vi "Main VERSION 1.1.vi"() -> ()   [LabVIEW 2017]
uses:
  <vilib>/Math Plots/3D Math Plots/3D Surface/3D Surface XCtrl/3D Surface.xctl
  <vilib>/Math Plots/3D Math Plots/3D Surface/3D Surface Datatype/3D Surface Datatype.lvclass
  CSV Reader Inputs.ctl
  Frequency_Type.ctl
  Measurement_Type.ctl
  Digital Channel Selector.ctl
  State.ctl
  Data.ctl
  <vilib>/Platform/TimedLoop/XDataNode/timing_clust.ctl
  <vilib>/Platform/TimedLoop/XDataNode/nitl_modes.ctl
  <vilib>/Platform/TimedLoop/XDataNode/wakeup.ctl
  <vilib>/addons/Control Design/_Model Construction/Data Typedefs.llb/CD DtoC Conversion Method.ctl
  <vilib>/imath/engines/lvmath2/RunTimeEngine/Managers/WorkSpace/UID Generator.vi
  <vilib>/imath/engines/lvmath2/RunTimeEngine/BuiltInFunctions/zpk_to_tf/NIMS_zpk_to_tf.vi
  <vilib>/imath/engines/lvmath2/RunTimeEngine/RunTimeType/NIMS_RunTimeType_From StrictType (excl LVString).vi
  <instcachedir>/0/NIMS_RunTimeType_From StrictType (excl LVString)_DC56D72BB6B948F98D63F1A957D87C42.lvgen/NIMS_RunTimeType_From StrictType (excl LVString)_DC56D72BB6B948F98D63F1A957D87C42_000.vi
  <vilib>/imath/engines/lvmath2/RunTimeEngine/ErrorHandling/NIMS_Error From Error Code.vi
  <vilib>/imath/engines/lvmath2/RunTimeEngine/LocalVariableDefStatement/MC_LocalVariableDefStatement_Display.vi
  <vilib>/imath/engines/lvmath2/RunTimeEngine/Managers/SymbolTable/Clear UID.vi
  <vilib>/imath/engines/lvmath2/RunTimeEngine/NodeEndStatement/NIMS_NodeEndStatement_Output.vi
  <instcachedir>/0/NIMS_NodeEndStatement_Output_53EC0D466D134D7ABD903AC30B43404B.lvgen/NIMS_NodeEndStatement_Output_53EC0D466D134D7ABD903AC30B43404B_005.vi
  <vilib>/imath/engines/lvmath2/RunTimeEngine/ErrorHandling/NIMS_Finalize Error.vi
  <vilib>/addons/Control Design/_Model Construction/Model Creation.llb/Model Creation SubVI/cd_Create Transfer Function Model.vi
  <vilib>/addons/Control Design/_Model Construction/Model Information.llb/Model Information SubVIs/cd_Set Names To TF Model.vi
  <vilib>/addons/Control Design/_Utility/Model Viewer.llb/Model Viewer SubVI/cd_Draw Transfer Function Equation (TF).vi
  <vilib>/addons/Control Design/_Time Response Analysis/Time Response.llb/Time Response subVI/cd_Linear Simulation (Transfer Function).vi
  <vilib>/addons/Control Design/_Dynamic Analysis/Dynamic Analysis.llb/Dynamic Analysis subVI/cd_Damping Ratio and Natural Frequency (Transfer Function).vi
  <vilib>/addons/Wavelet Analysis/application.llb/WA Detrend (Waveform).vi
  Program Files (x86)/National Instruments/LabVIEW 2017/vi.lib/addons/System Identification/Data Preprocess.llb/SI Lowpass Filter (SISO Waveform).vi
  <vilib>/addons/Time Series Analysis/Modeling and Prediction.llb/TSA ARMA Modeling (Waveform).vi
  <vilib>/addons/Control Design/_Model Conversions/Continuous and Discrete.llb/Continuous and Discrete SubVI/cd_Convert Discrete to Continuous (TF).vi
  <vilib>/addons/Control Design/_Model Conversions/Model Type.llb/Model Conversion SubVI/cd_Convert Transfer Function to State-Space Model.vi
  <vilib>/addons/Control Design/_Dynamic Analysis/Dynamic Analysis.llb/Dynamic Analysis subVI/cd_Damping Ratio and Natural Frequency (State-Space).vi
  <vilib>/imath/engines/lvmath2/RunTimeEngine/BuiltInFunctions/sort/NIMS_[2o]_sort(RRowV,I32,Str).vi
  <instcachedir>/0/NIMS_[2o]_sort(RRowV,I32,Str)_E84E23B068DF4763991B1E74560868DE.lvgen/NIMS_[2o]_sort(RRowV,I32,Str)_E84E23B068DF4763991B1E74560868DE_000.vi
  <vilib>/imathl/engines/lvmath/Functions/Error Handling/Create Error.vi
  <vilib>/imath/engines/lvmath2/RunTimeEngine/IndexRead/NIMS V(V).vi
  <instcachedir>/0/NIMS V(V)_298D9CB7BFEB42B8BC8D9C3C28AE8C70.lvgen/NIMS V(V)_298D9CB7BFEB42B8BC8D9C3C28AE8C70_000.vi
  <instcachedir>/0/NIMS V(V)_298D9CB7BFEB42B8BC8D9C3C28AE8C70.lvgen/NIMS V(V)_298D9CB7BFEB42B8BC8D9C3C28AE8C70_001.vi
  <vilib>/imath/engines/lvmath2/RunTimeEngine/BitwiseOperatorToken/NIMS_Bitwise_Operator_And.vi
  <instcachedir>/0/NIMS_Bitwise_Operator_And_BF79565AECDF4B89921EA9614C6BB008.lvgen/NIMS_Bitwise_Operator_And_BF79565AECDF4B89921EA9614C6BB008_001.vi
  <vilib>/imath/engines/lvmath2/RunTimeEngine/BuiltInFunctions/imag/NIMS_imag(Complex).vi
  <instcachedir>/0/NIMS_imag(Complex)_3180D40D00C843A49C2B33397F857BF3.lvgen/NIMS_imag(Complex)_3180D40D00C843A49C2B33397F857BF3_002.vi
  <vilib>/imath/engines/lvmath2/RunTimeEngine/BuiltInFunctions/findnz/NIMS_[1o]_findnz(GRowV).vi
  <instcachedir>/0/NIMS_[1o]_findnz(GRowV)_4566141FE5BA40B7B10E18ED0AB78B2D.lvgen/NIMS_[1o]_findnz(GRowV)_4566141FE5BA40B7B10E18ED0AB78B2D_000.vi
  <vilib>/imath/engines/lvmath2/RunTimeEngine/ErrorHandling/NIMS_Create Error From Enums.vi
  <instcachedir>/0/NIMS_NodeEndStatement_Output_53EC0D466D134D7ABD903AC30B43404B.lvgen/NIMS_NodeEndStatement_Output_53EC0D466D134D7ABD903AC30B43404B_000.vi
  <vilib>/addons/Time Series Analysis/Correlation and Spectral Analysis.llb/TSA ARMA Spectrum (Waveform).vi
  <vilib>/imath/engines/lvmath2/RunTimeEngine/RangeToken/NIMS_Range.vi
  <instcachedir>/0/NIMS_Range_8C005833F4504FD4A29AA23D6150121A.lvgen/NIMS_Range_8C005833F4504FD4A29AA23D6150121A_000.vi
  <vilib>/imath/engines/lvmath2/RunTimeSupport/NIMS_Error if Not Equal.vi
  <instcachedir>/0/NIMS_Error if Not Equal_E5646C1EFB50404BB0542B8CFB81CE27.lvgen/NIMS_Error if Not Equal_E5646C1EFB50404BB0542B8CFB81CE27_001.vi
  <instcachedir>/0/NIMS_Error if Not Equal_E5646C1EFB50404BB0542B8CFB81CE27.lvgen/NIMS_Error if Not Equal_E5646C1EFB50404BB0542B8CFB81CE27_000.vi
  <vilib>/imath/engines/lvmath2/RunTimeEngine/IndexRead/NIMS V($).vi
  <instcachedir>/0/NIMS V($)_C593F32C7F6B43C7B1793952E292524F.lvgen/NIMS V($)_C593F32C7F6B43C7B1793952E292524F_001.vi
  <vilib>/imath/engines/lvmath2/RunTimeEngine/IndexReplace/NIMS M(S,$)=V.vi
  <instcachedir>/0/NIMS M(S,$)=V_552265ADF67C4F4FB07E91CD22492551.lvgen/NIMS M(S,$)=V_552265ADF67C4F4FB07E91CD22492551_000.vi
  <vilib>/imath/engines/lvmath2/RunTimeEngine/IndexReplace/NIMS V(S)=S.vi
  <instcachedir>/0/NIMS V(S)=S_EDDEB2B900FD4B108B325BCE58B17C3D.lvgen/NIMS V(S)=S_EDDEB2B900FD4B108B325BCE58B17C3D_000.vi
  <vilib>/imath/engines/lvmath2/RunTimeEngine/IndexReplace/NIMS V(V)=V.vi
  <instcachedir>/0/NIMS V(V)=V_ACB9F458E2974419B362D656D10048D7.lvgen/NIMS V(V)=V_ACB9F458E2974419B362D656D10048D7_000.vi
  <vilib>/imath/engines/lvmath2/RunTimeEngine/IndexRead/NIMS M(V,$).vi
  <instcachedir>/0/NIMS M(V,$)_21A5155762F74C04AE4EA67BEE0D3EF5.lvgen/NIMS M(V,$)_21A5155762F74C04AE4EA67BEE0D3EF5_004.vi
  <instcachedir>/0/NIMS_NodeEndStatement_Output_53EC0D466D134D7ABD903AC30B43404B.lvgen/NIMS_NodeEndStatement_Output_53EC0D466D134D7ABD903AC30B43404B_009.vi
  <instcachedir>/0/NIMS_NodeEndStatement_Output_53EC0D466D134D7ABD903AC30B43404B.lvgen/NIMS_NodeEndStatement_Output_53EC0D466D134D7ABD903AC30B43404B_002.vi
  <instcachedir>/0/NIMS_NodeEndStatement_Output_53EC0D466D134D7ABD903AC30B43404B.lvgen/NIMS_NodeEndStatement_Output_53EC0D466D134D7ABD903AC30B43404B_001.vi
  <vilib>/Math Plots/3D Math Plots/3D Surface/3D Surface Datatype/Public/Plot Helper (Vector).vi
  <vilib>/platform/TimedLoop/XDataNode/XDataNode.xnode
  Program Files (x86)/National Instruments/LabVIEW 2017/vi.lib/addons/System Identification/NI_SysID.lvlib
  <vilib>/addons/_Advanced Signal Processing/NI_AdvSigProcWA.lvlib
  <vilib>/addons/_Advanced Signal Processing/NI_AdvSigProcTSA.lvlib
  <vilib>/addons/Control Design/_Model Construction/NI_LinSys_Model Creation.lvlib
  <vilib>/addons/Control Design/_Model Conversions/NI_CD_Continuous and Discrete.lvlib
  <vilib>/addons/Control Design/_Model Construction/NI_LinSys_Data Typedefs.lvlib
  <vilib>/Analysis/NI_AALBase.lvlib
  <vilib>/addons/Control Design/_Dynamic Analysis/NI_CD_Dynamic Analysis.lvlib
  <vilib>/Platform/TimedLoop/XDataNode/XDNodeRunTimeDep.lvlib
  <vilib>/addons/Control Design/_Model Conversions/NI_CD_Model Type.lvlib
  <vilib>/Analysis/NI_AALPro.lvlib
  <vilib>/addons/Control Design/_Time Response Analysis/NI_CD_Time Response.lvlib
  <vilib>/imath/engines/lvmath2/RunTimeEngine/Managers/SymbolTable/NIMS_WorkSpace.lvlib
  <vilib>/addons/Control Design/_Model Construction/NI_LinSys_Model Information.lvlib
  <vilib>/addons/Control Design/_Utility/NI_CD_Model Viewer.lvlib
  <vilib>/S3DK/PMU Recorder Light/PMU Recorder Light.lvlib
panel:
  in  "Tab Control 3":enum32{"Test", "Simulation"}(tab)
  in  "Terminal ID 2 (Phase Comparison)":dbl
  in  "Test Method":enum16{"Use PRL Data", "Read from CSV File"}(ring)
  in  "CSV Reader Inputs":T1={"Frequency Type"=enum."Frequency", "Measurement Type"=enum."Power", "Digital Channel Selector"=enum."2", "OGE Type"=enum."OGnE", "CSV File Input"=path ""}
  in  "Terminal ID":dbl
  in  "Input Poles":cdb[](array[numeric])
  in  "Input Zeros":cdb[](array[numeric])
  out "Input Transfer Function":picture
  in  "Input Frequency (Hz)":dbl
  in  "Input Damping Ratio (%)":dbl
  in  "Simulation Method":T5(ring)
  out "Poles":cdb[](array[numeric]) format="%.2f"
  out "Damping Ratios (%)":dbl[](array[numeric]) format="%.2f"
  out "Natural Frequencies":dbl[](array[numeric]) format="%.2f"
  in  "Tab Control":enum32{"Data", "Preprocessed Data"}(tab)
  out "Real-time data":waveform(dbl)(graph)={"t0"=timestamp(3467964116.0127993 s since 1904-01-01), "dt"=0.02, "Y"=array[30000 elements]}
  out "Preprocessed data":waveform(dbl)(graph)={"t0"=timestamp(3467964116.0127993 s since 1904-01-01), "dt"=0.2, "Y"=array[3000 elements]}
  in  "Tab Control 2":T6(tab)=enum."Options"
  out "Critical Damping [%]":dbl
  out "Critical Frequency [Hz]":dbl
  out "Estimated Complex Plane":cluster{dbl[], dbl[]}(graph)
  out "Damping ratio evolution":dbl[][](graph)
  in  "Number of critical modes":i32=1
  in  "Length of Spectra [s]":dbl=12.0
  out "Spectrogram":refnum<class "3D Plot Datatype.lvclass">[](xcontrol)
  in  "dB Scale":bool=TRUE
  out "Spectrum":cluster{"f0":dbl, "df":dbl, "S(f)":dbl[]}(graph)={"f0"=0.0, "df"=0.0048828125, "S(f)"=[]}
  out "ARMA Transfer Function":picture
  out "Picture 9":picture
  out "Picture 8":picture
  out "Picture 7":picture
  out "Picture 6":picture
  out "Picture 5":picture
  out "Picture 4":picture
  out "Picture 3":picture
  out "Picture 2":picture
  out "Picture 1":picture
  out "Std of Damping":dbl[](array[numeric])=[3.167813045881809]
  out "Mean Damping [%]":dbl[](array[numeric])=[5.49924934647624]
  out "Frequency[Hz]":dbl[](array[numeric])=[1.626086044993813, 0.5198061588603065, 1.9739015777045272] format="%.4f"
  out "Damping Ratio [%]":dbl[](array[numeric])=[11.530156484123282, 15.381771713903165, 15.639879258359347] format="%.4f"
  out "Complex Poles":cdb[](array[numeric])=[-1.1780360817698377+10.148858009104277i, -0.5023745738423925+3.227170083530164i, -1.9397187258807729+12.249765461704891i] format="%.4f"
  in  "Upper Damping [%]":dbl=20.0
  in  "Lower Damping [%]":dbl
  in  "Upper Frequency [Hz]":dbl=2.0
  in  "Lower Frequency [Hz]":dbl=0.08
  in  "Signal Selection":T7(radio)=enum."Analog"
  in  "Downsampling Ratio":dbl=1.0
  in  "LPF Cut-off Frequency [Hz]":dbl=2.5
  in  "Low-Pass Filter Order":i32=5
  in  "Detrend Cut-off Frequency (Hz)":dbl=0.05
  in  "MA Order":i32=10
  in  "Sampling Frequency (Hz)":dbl=50.0
  in  "AR Order":i32=25
  in  "Parcel Length (Simulation)":i32=30000
  in  "Refresh Rate [s]":i32=10
  in  "Std Threshold":dbl=1.35
  out "Parcel Length (SDK or Simulation)":i32=30000
  in  "Simulate Data?":bool
  out "Simulation":bool
  in  "stop":bool
  # "Simulated Expected Values"
  # "**Must enter CSV file before running"
  # "***Has the ability to shows more than 1 graph based on parameters\n\n- Each row of data (numerical results) equates to 1 mode"
  # "MA\n_______\n\n   AR"
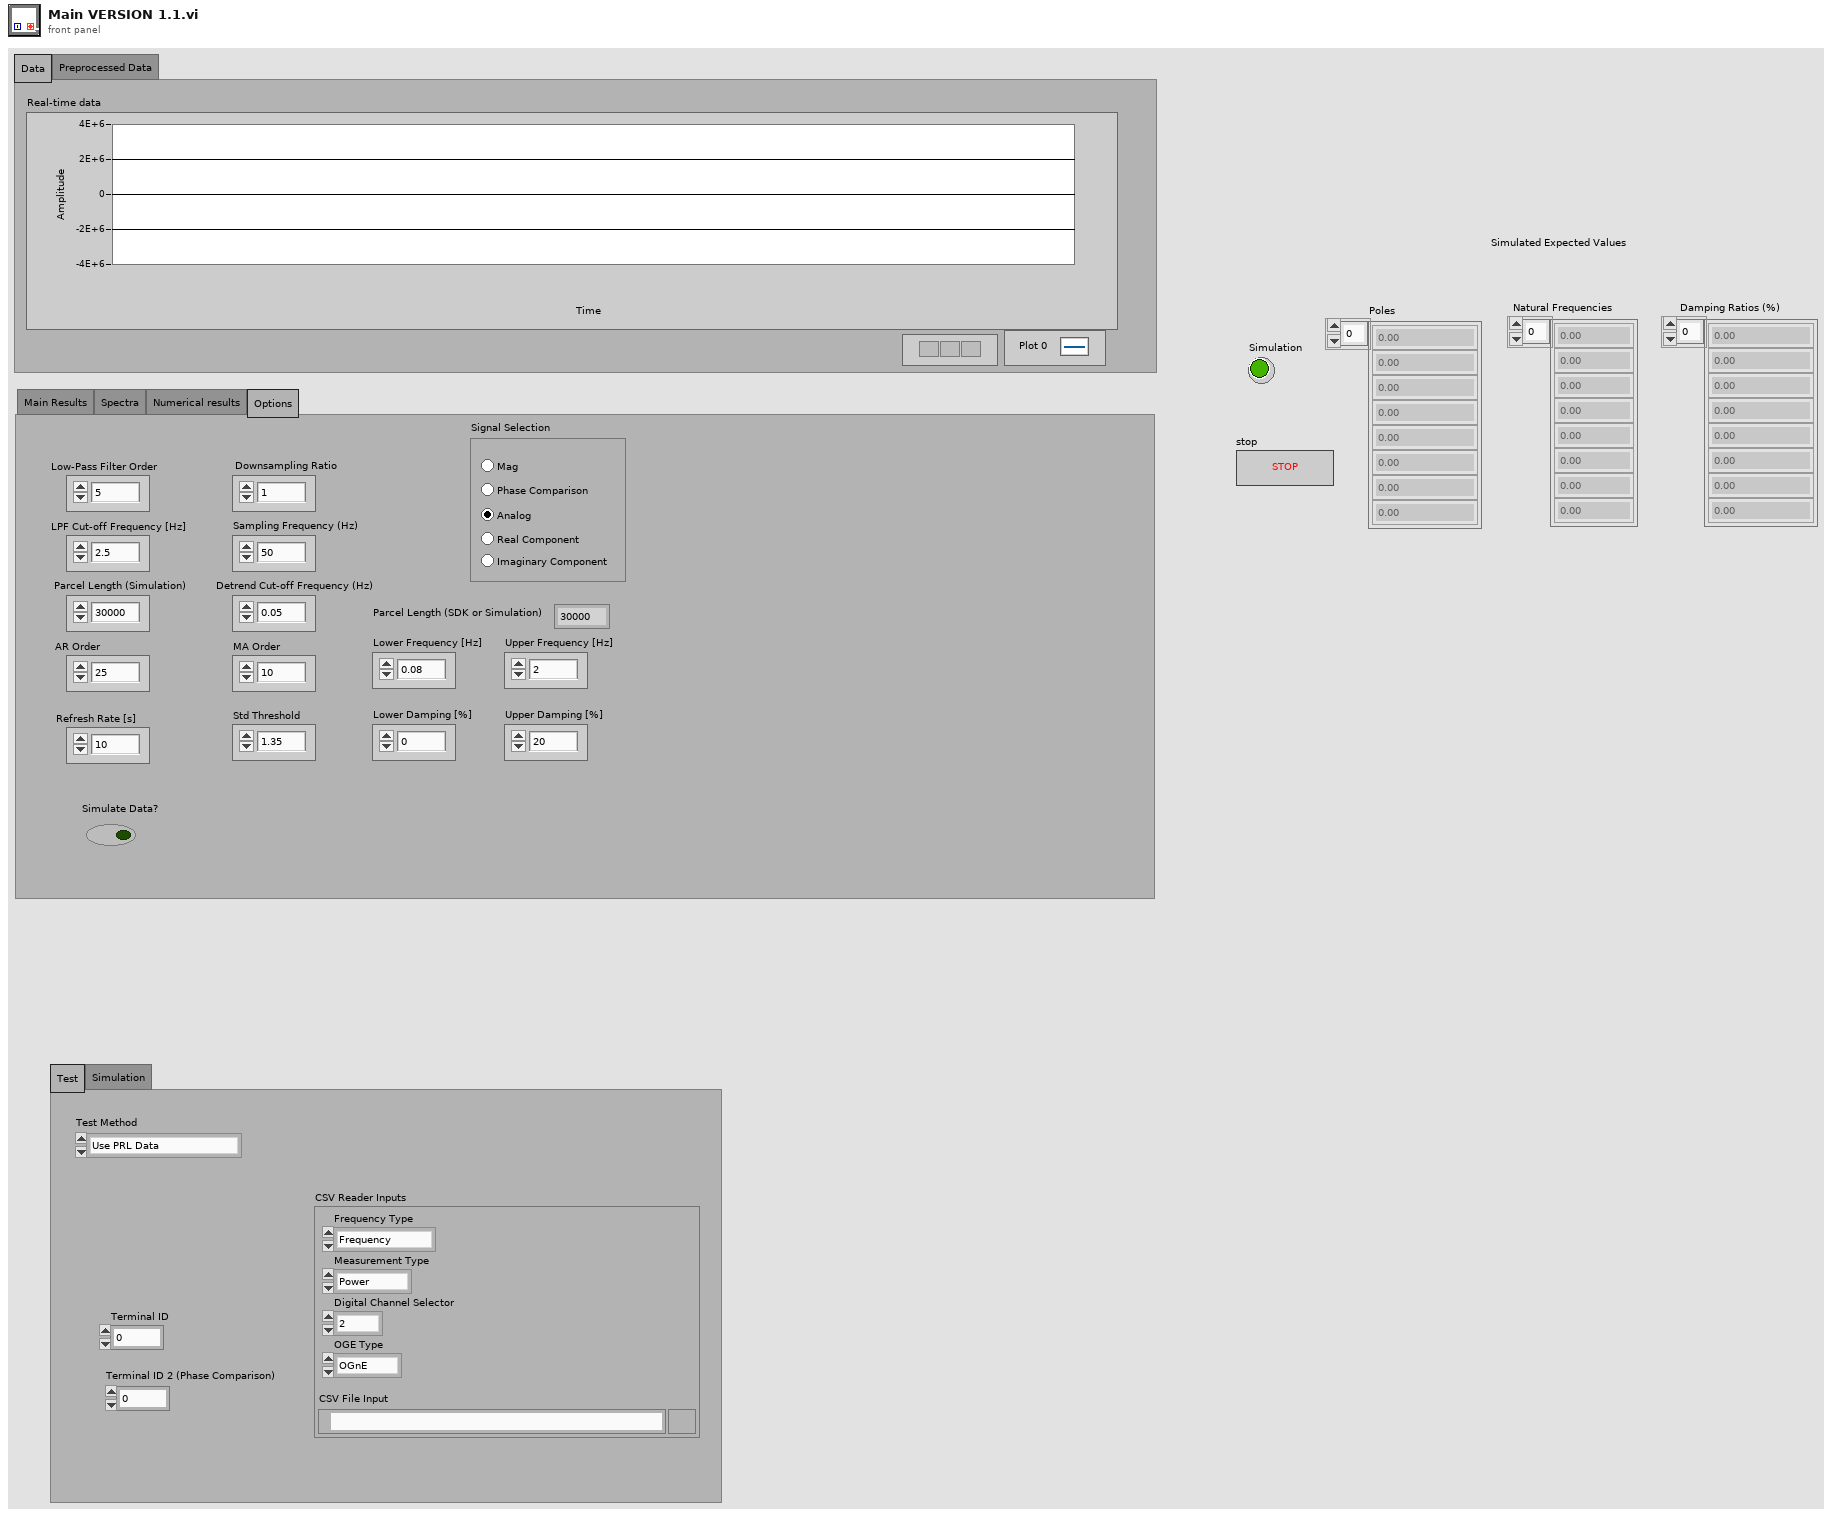
[diagram p1: front panel]
types:
  T1 = typedef "CSV Reader Inputs.ctl" = cluster{"Frequency Type":T2, "Measurement Type":T3, "Digital Channel Selector":T4, "OGE Type":enum16{"WAN OGE", "OGnE"}, "CSV File Input":path}
  T2 = typedef "Frequency_Type.ctl" = enum16{"Frequency", "df/dt"}
  T3 = typedef "Measurement_Type.ctl" = enum16{"Voltage", "Current", "Power"}
  T4 = typedef "Digital Channel Selector.ctl" = enum16{"1", "2", "3"}
  T5 = enum16{"Use Input Frequency/D.R.", "Use Input Poles/Zeroes"}
  T6 = enum32{"Main Results", "Spectra", "Numerical results", "Options"}
  T7 = enum32{"Mag", "Phase", "Analog", "Real Component", "Imaginary Component"}
  T8 = enum8{"Enabled", "Disabled", "Disabled and Grayed Out"}
  T9 = typedef "data.ctl" = cluster{"Waveform":waveform(dbl), "Parcel Length":i32, "AR Order":i32, "Sampling Frequency":dbl, "MA Order ":i32}
  T10 = typedef "State.ctl" = enum16{"Initialize", "Read Real Data", "Read Simulated Data", "Preprocessing", "Compute AR/MA Coeffs", "Get Spectrum"}
  T11 = typedef "XDNodeRunTimeDep.lvlib/timing_clust.ctl" = cluster{"Expected End [f-1]":u64, "Actual End [f-1]":u64, "Finished Late? [f-1]":bool, "Expected End [i-1]":u64, "Actual End [i-1]":u64, "Finished Late? [i-1]":bool, "Expected Start [i]":u64, "Actual Start [i]":u64, "Expected Start [f]":u64, "Actual Start [f]":u64, "Source Name":string, "Structure Name":string, "Period":i64, "Deadline":i64, "Offset":i64, "Start":i64, "Priority":i32, "Timeout":i32, "Mode":T12, "Wakeup Reason":T13, "Error":errorcluster, "Source Type":string, "Secondary Source Type":string, "Global End Time":u64, "Global Start Time":u64, "Frame Duration":u64, "Iteration Duration":u64, "Assigned CPU":i32, "I/O Scan Engine Mode":u32}
  T12 = typedef "XDNodeRunTimeDep.lvlib/nitl_modes.ctl" = enum32{"No Change", "Process missed periods, maintain original phase", "Discard missed periods, maintain original phase", "Process missed periods, ignore original phase", "Discard missed periods, ignore original phase"}
  T13 = typedef "XDNodeRunTimeDep.lvlib/wakeup.ctl" = enum32{"Normal", "Aborted", "Asynchronous wakeup", "Timing source error", "Timed loop error", "Timeout"}
  T14 = typedef "Terminal Data.ctl" = cluster{"Terminal Name":string, "Terminal ID":dbl, "Timestamps":timestamp[], "Phasor Data":cdb[], "Analog Data":dbl[], "Status":dbl[], "Digital Data":dbl[]}
  T15 = typedef "NI_LinSys_Model Typedefs.lvlib/CD Transfer Function Model (MIMO).ctl" = cluster{"properties":T16, "transfer function(s)":T17[][]}
  T16 = typedef "NI_LinSys_Model Typedefs.lvlib/CD General Elements.ctl" = cluster{"Model name":string, "Input names":string[], "Output names":string[], "Input Delays":dbl[], "Output Delays":dbl[], "Sampling Time":dbl, "Notes":string}
  T17 = typedef "NI_LinSys_Model Typedefs.lvlib/CD Transfer Function Model (SISO).ctl" = cluster{"Numerator":dbl[], "Denominator":dbl[], "delay":dbl}
  T18 = typedef "NI_LinSys_Data Typedefs.lvlib/CD MIMO Time Response Data.ctl" = cluster{"Time":dbl[], "Outputs Data":dbl[][][], "States Data":dbl[][][], "plot type":T19}
  T19 = typedef "NI_LinSys_Data Typedefs.lvlib/CD Plot Types Enum.ctl" = enum16{"bode-magnitude", "bode-phase", "nichols", "nyquist", "singular values", "step", "impulse", "initial", "simulation", "nyquist with separation"}
  T20 = typedef "NI_LinSys_Data Typedefs.lvlib/CD DtoC Conversion Method.ctl" = u16
  T21 = typedef "NI_LinSys_Model Typedefs.lvlib/CD State Space Model (MIMO).ctl" = cluster{"properties":T16, "A":dbl[][], "B":dbl[][], "C":dbl[][], "D":dbl[][], "StateNames":string[], "Transport Delay":dbl[][]}
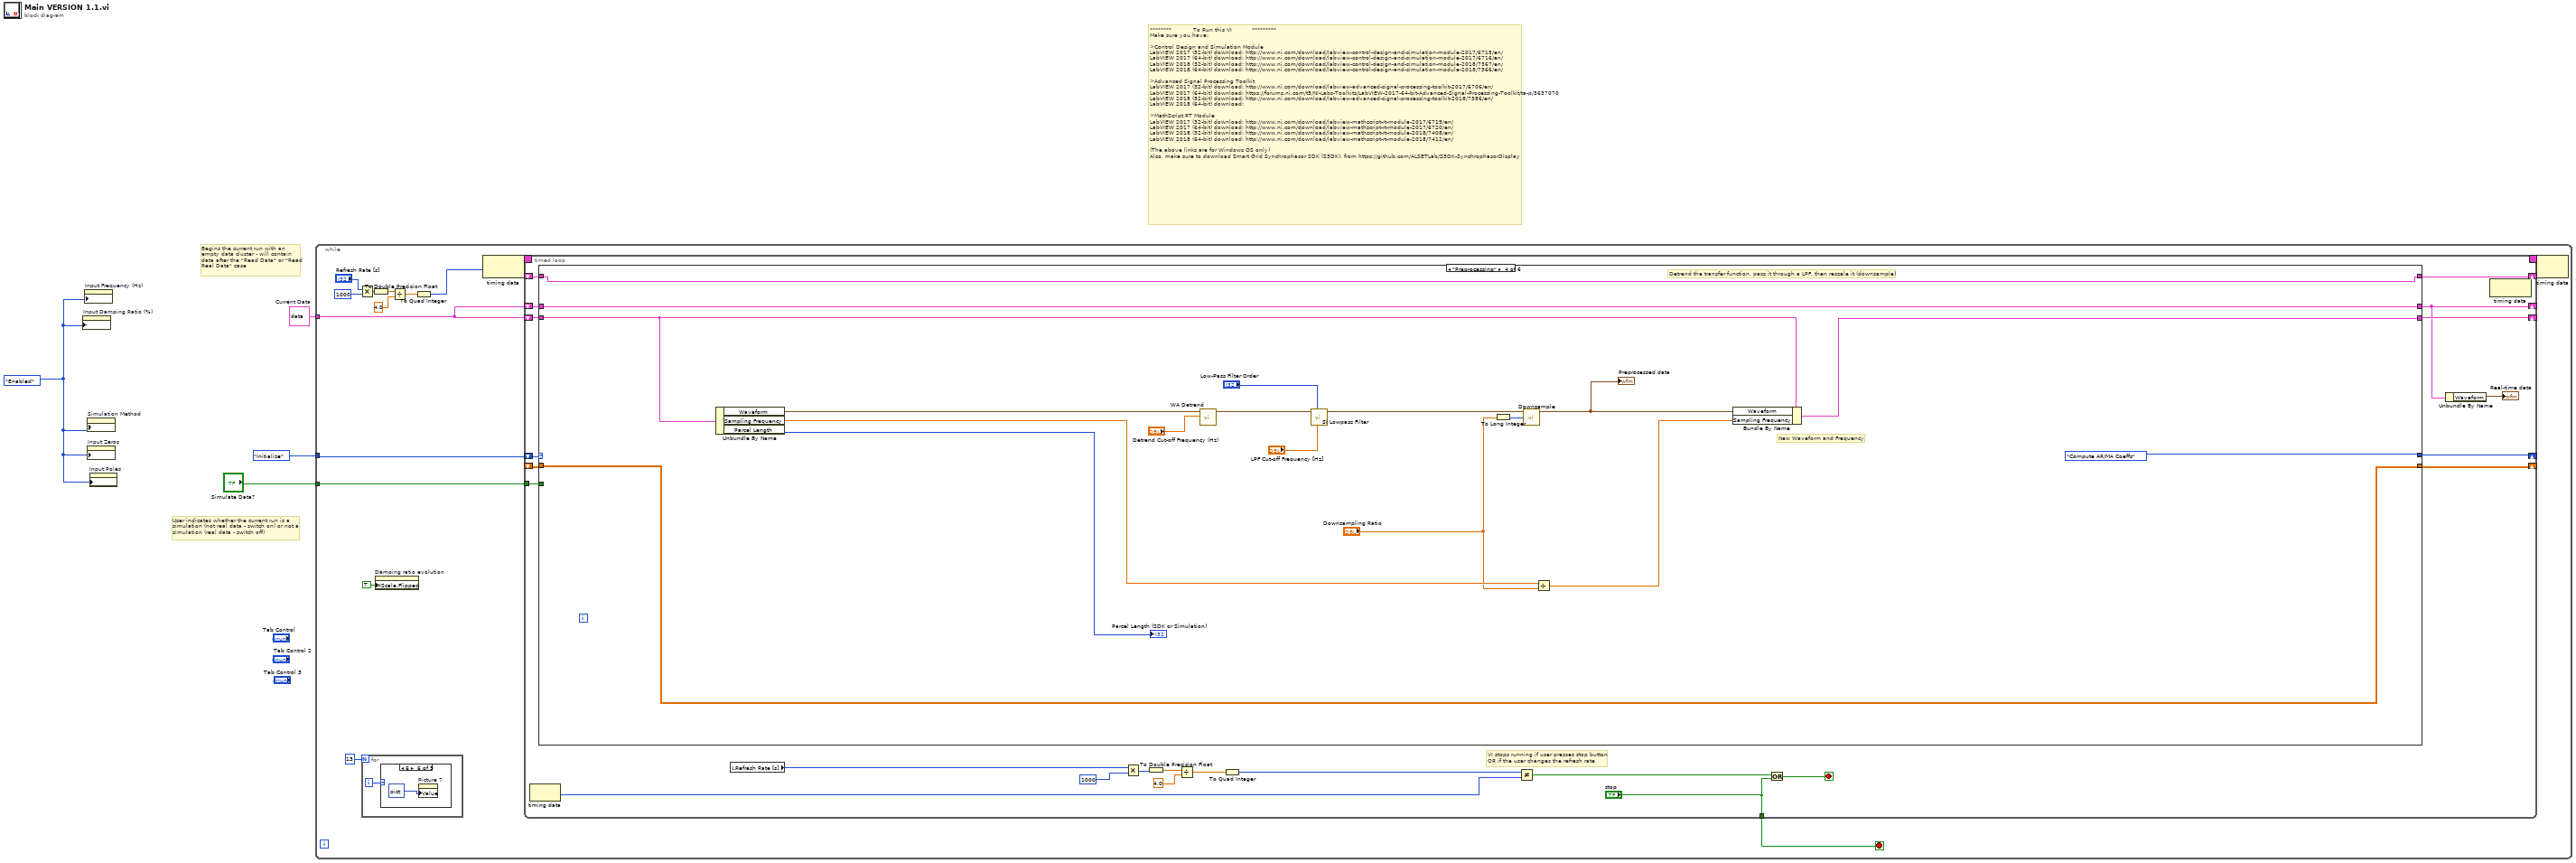
[diagram p0: block diagram]
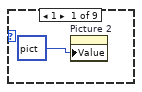
[diagram p2: hidden frame]
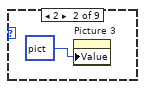
[diagram p3: hidden frame]
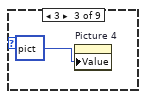
[diagram p4: hidden frame]
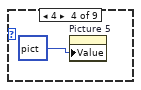
[diagram p5: hidden frame]
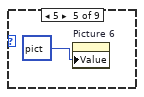
[diagram p6: hidden frame]
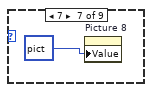
[diagram p7: hidden frame]
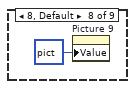
[diagram p8: hidden frame]
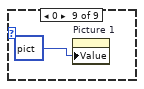
[diagram p9: hidden frame]
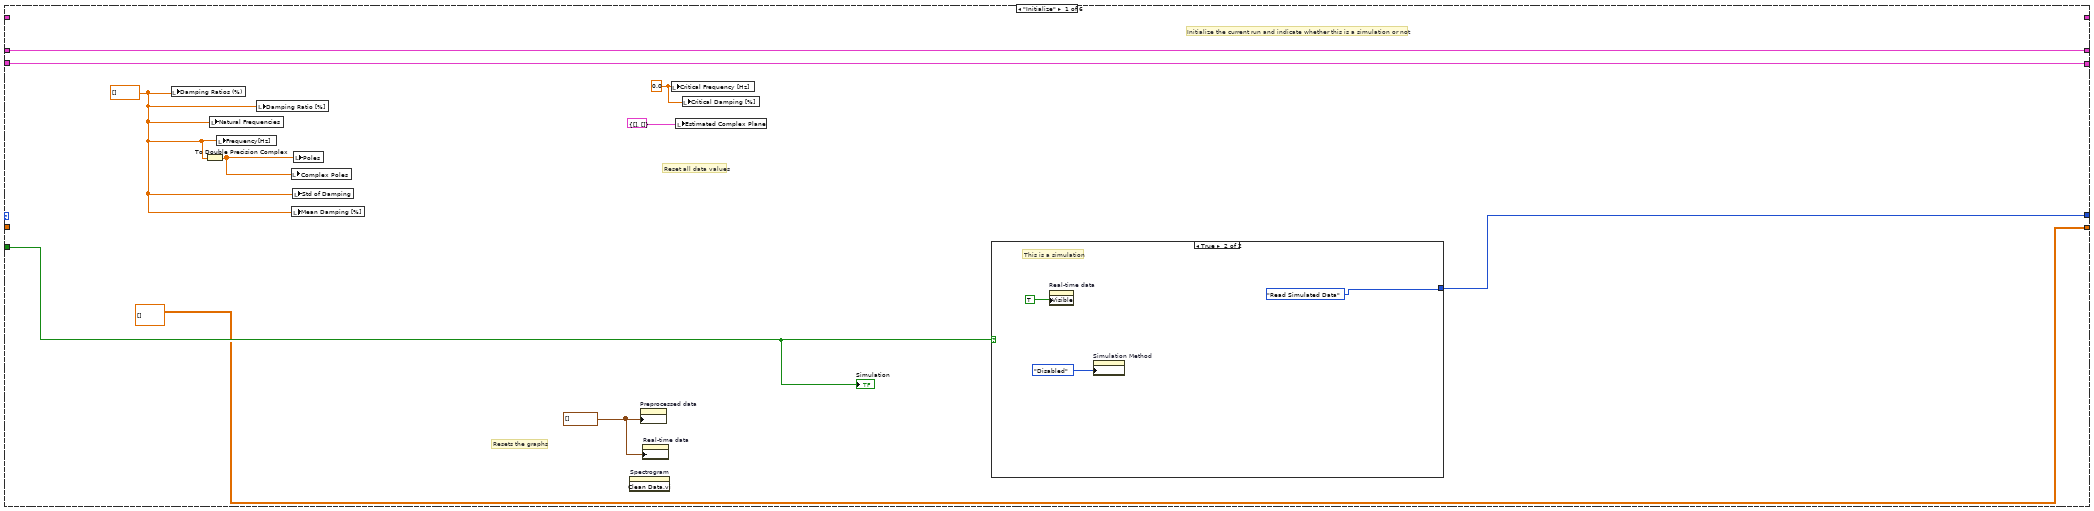
[diagram p10: hidden frame]
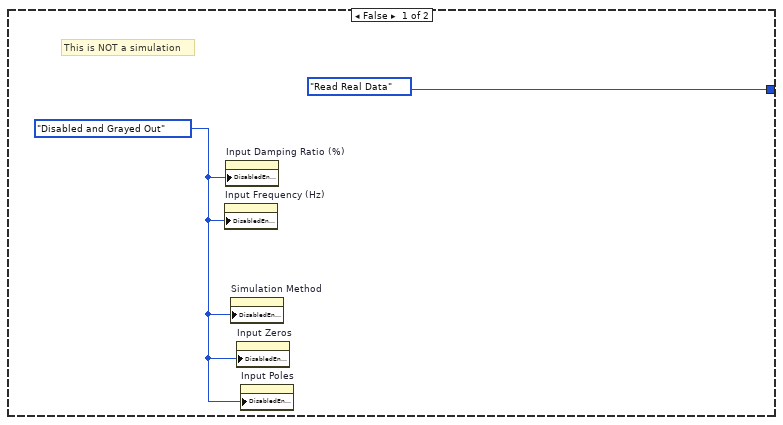
[diagram p11: hidden frame]
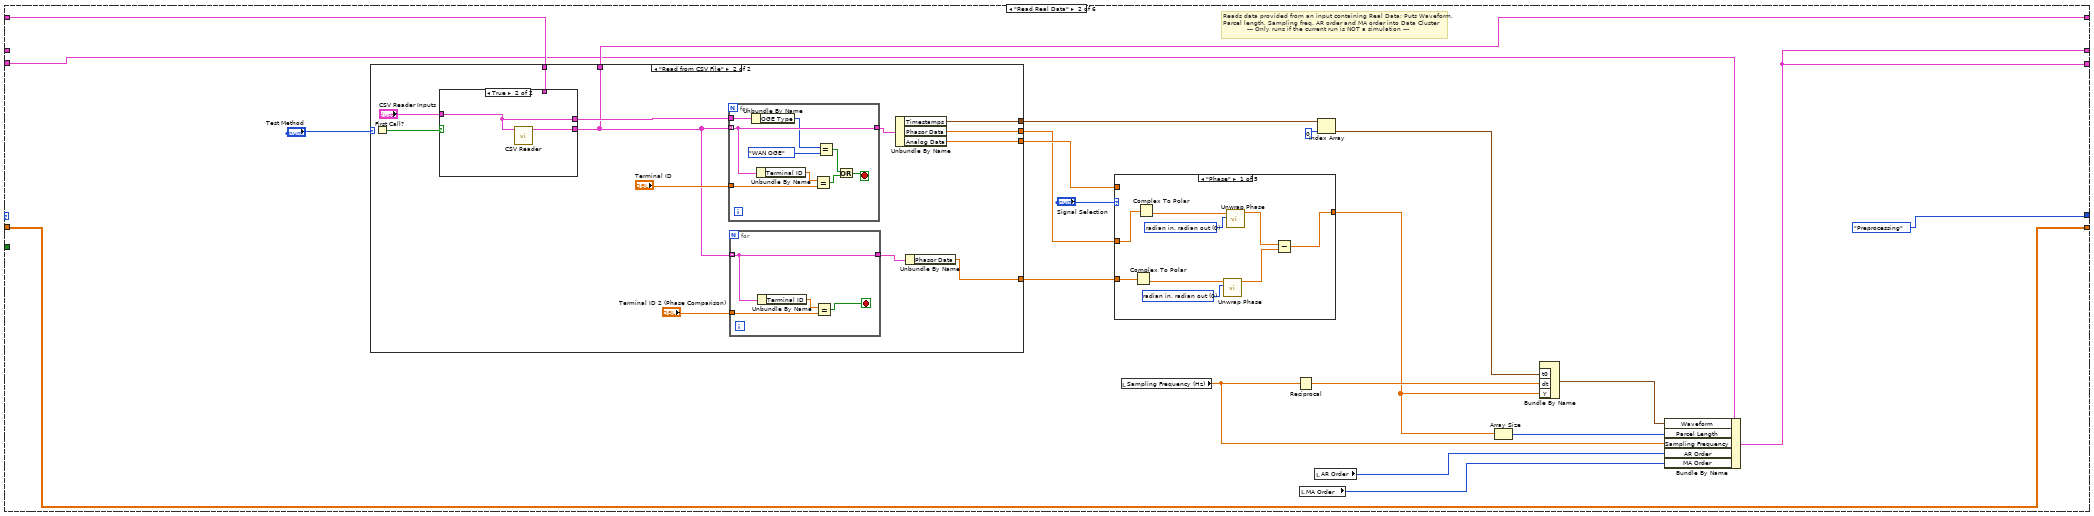
[diagram p12: hidden frame]
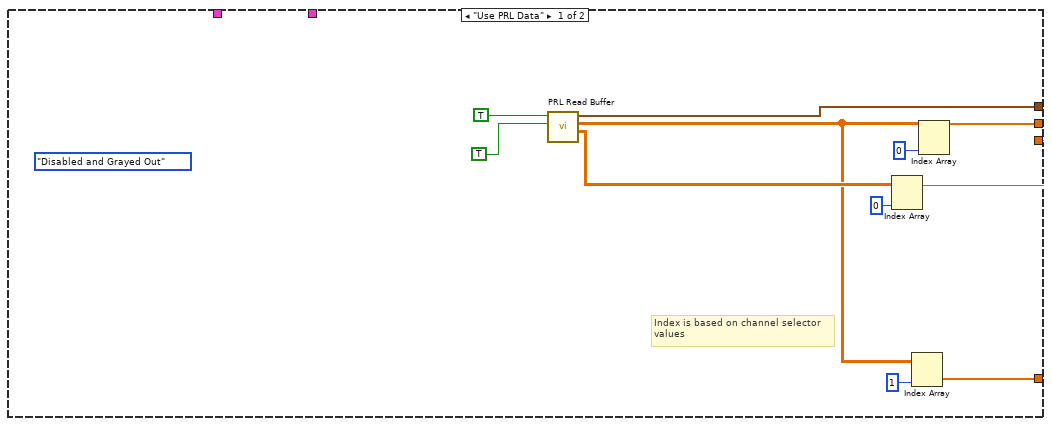
[diagram p13: hidden frame]
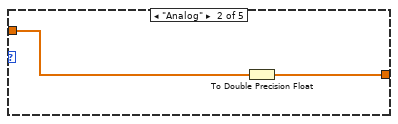
[diagram p15: hidden frame]
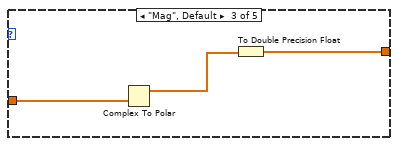
[diagram p16: hidden frame]
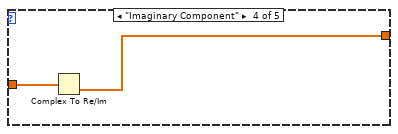
[diagram p17: hidden frame]
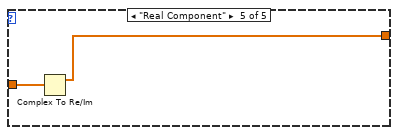
[diagram p18: hidden frame]
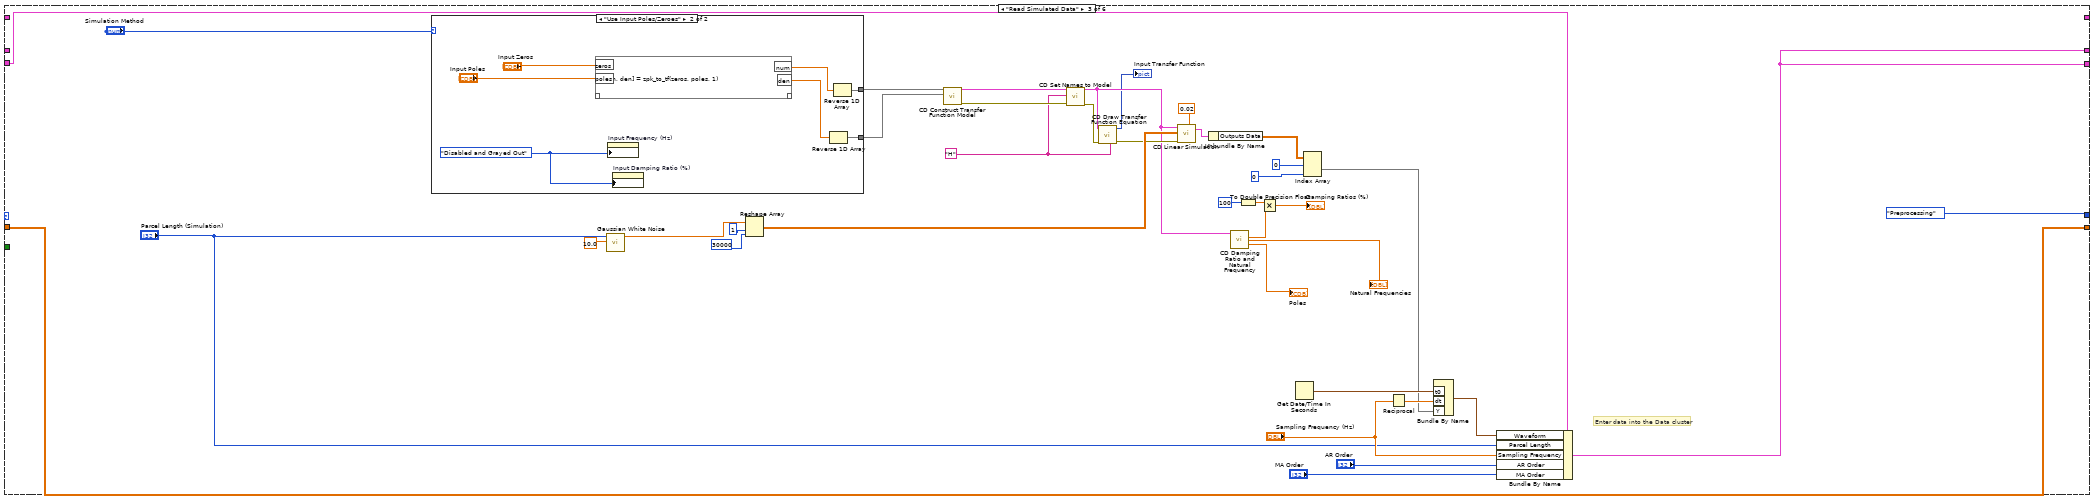
[diagram p19: hidden frame]
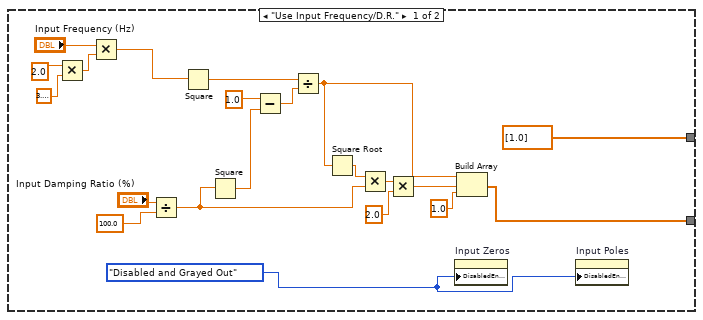
[diagram p20: hidden frame]
diagram:
  w2 = T8."Enabled" ("Disabled")
  w3 = T9 {"Waveform"={"t0"=timestamp(0 s since 1904-01-01), "dt"=1.0, "Y"=[]}, "Parcel Length"=0, "AR Order"=0, "Sampling Frequency"=0.0, "MA Order "=0}  # Current Data
  # "Begins the current run with an \nempty data cluster - will contain\ndata after the \"Read Data\" or \"Read \nReal Data\" case"
  # "User indicates whether the current run is a \nsimulation (not real data - switch on) or not a\nsimulation (real data - switch off)"
  # "********            To Run this VI           *********\nMake sure you have:\n\n>Control Design and Simulation Module\nLabVIEW 2017 (32-bit) download: http://www.ni.com/download/labview-control-design-and-simulation-module-2017/6715/en/\nLabVIEW 2017 (64-bit) download: http://www.ni.com/download/labview-control-design-and-simulation-module-2017/6716/en/ \nLabVIEW 2018 (32-bit) download: http://www.ni.com/download/labview-control-design-and-simulation-module-2018/7367/en/\nLabVIEW 2018 (64-bit) download: http://www.ni.com/download/labview-control-design-and-simulation-module-2018/7366/en/\n\n>Advanced Signal Processing Toolkit\nLabVIEW 2017 (32-bit) download: http://www.ni.com/download/labview-advanced-signal-processing-toolkit-2017/6706/en/\nLabVIEW 2017 (64-bit) download: https://forums.ni.com/t5/NI-Labs-Toolkits/LabVIEW-2017-64-bit-Advanced-Signal-Processing-Toolkit/ta-p/3637070\nLabVIEW 2018 (32-bit) download: http://www.ni.com/download/labview-advanced-signal-processing-toolkit-2018/7386/en/\nLabVIEW 2018 (64-bit) download:\n\n>MathScript RT Module\nLabVIEW 2017 (32-bit) download: http://www.ni.com/download/labview-mathscript-rt-module-2017/6719/en/\nLabVIEW 2017 (64-bit) download: http://www.ni.com/download/labview-mathscript-rt-module-2017/6720/en/ \nLabVIEW 2018 (32-bit) download: http://www.ni.com/download/labview-mathscript-rt-module-2018/7408/en/\nLabVIEW 2018 (64-bit) download: http://www.ni.com/download/labview-mathscript-rt-module-2018/7412/en/ \n\n(The above links are for Windows OS only)\nAlso, make sure to download Smart Grid Synchrophasor SDK (S3DK), from https://github.com/ALSETLab/S3DK-SynchrophasorDisplay"
  n1 = property on="Input Damping Ratio (%)" class="DigNum (strict)"("DisabledEnum"=w2) -> ()  [unwired: 2 in, 2 out]
  n2 = property on="Input Frequency (Hz)" class="DigNum (strict)"("DisabledEnum"=w2) -> ()  [unwired: 2 in, 2 out]
  n3 = property on="Simulation Method" class="Enum (strict)"("DisabledEnum"=w2) -> ()  [unwired: 2 in, 2 out]
  n4 = property on="Input Zeros" class="Arr (strict)"("DisabledEnum"=w2) -> ()  [unwired: 2 in, 2 out]
  n5 = property on="Input Poles" class="Arr (strict)"("DisabledEnum"=w2) -> ()  [unwired: 2 in, 2 out]
  n6 = while {
    tunnel: State."Initialize" ("Enum") -> [w5]
    tunnel: w3 -> [w6]
    tunnel: "Simulate Data?" -> [w10]
    stop <- w12 stop-if-true
    n7 = Multiply(x="Refresh Rate [s]", y=1000) -> (x*y=w7:i32)
    n8 = for {
      N: 13 -> [_]
      i -> [w20]
      n9 = case shown="6" w20 {
        frame 1 {
          n10 = property on="Picture 2" class="Pict"("Value"=picture bytes[260130] ("Picture 9")) -> ()  [unwired: 2 in, 2 out]
        }
        frame 2 {
          n11 = property on="Picture 3" class="Pict"("Value"=picture bytes[260130] ("Picture 9")) -> ()  [unwired: 2 in, 2 out]
        }
        frame 3 {
          n12 = property on="Picture 4" class="Pict"("Value"=picture bytes[260130] ("Picture 9")) -> ()  [unwired: 2 in, 2 out]
        }
        frame 4 {
          n13 = property on="Picture 5" class="Pict"("Value"=picture bytes[260130] ("Picture 9")) -> ()  [unwired: 2 in, 2 out]
        }
        frame 5 {
          n14 = property on="Picture 6" class="Pict"("Value"=picture bytes[260130] ("Picture 9")) -> ()  [unwired: 2 in, 2 out]
        }
        frame 6 {
          n15 = property on="Picture 7" class="Pict"("Value"=picture bytes[260130] ("Picture 9")) -> ()  [unwired: 2 in, 2 out]
        }
        frame 7 {
          n16 = property on="Picture 8" class="Pict"("Value"=picture bytes[260130] ("Picture 9")) -> ()  [unwired: 2 in, 2 out]
        }
        frame 8, Default {
          n17 = property on="Picture 9" class="Pict"("Value"=picture bytes[260130] ("Picture 9")) -> ()  [unwired: 2 in, 2 out]
        }
        frame 0 {
          n18 = property on="Picture 1" class="Pict"("Value"=picture bytes[260130] ("Picture 9")) -> ()  [unwired: 2 in, 2 out]
        }
      }
    }
    n19 = To Double Precision Float(number=w7) -> (double precision float=w8:dbl)
    n20 = property on="Damping ratio evolution" class="WFGraph (strict)"("XScale.Flipped"=TRUE ("X Scale.Flipped")) -> ()  [unwired: 2 in, 2 out]
    n21 = Divide(x=w8, y=4.0) -> (x/y=w14:dbl)
    n22 = To Quad Integer(1:w14) -> (0:w13:i64)
    n23 = node-c288(w13) -> (w19:T11)
    n24 = timed-loop {
      shift-right: [w39] -> _
      shift-left: w6 -> [w52]
      shift-right: [w32] -> _
      shift-left: w5 -> [w33]
      timing: w19 -> [_]
      timing-out: [_] -> w18
      tunnel: ["stop"] -> w12
      shift-right: [w42] -> _
      shift-left: _ -> [w41]
      tunnel: w10 -> [w40]
      shift-right: [w37] -> _
      shift-left: w6 -> [w36]
      shift-right: [w31] -> _
      shift-left: _ -> [w30]
      stop <- w51 stop-if-true
      # "VI stops running if user presses stop button\nOR if the user changes the refresh rate"
      n25 = node-c288() -> (w50:i64)  [unwired: 1 in]
      n26 = case shown="\"Preprocessing\"" w33 {
        tunnel: w52 -> [w65 w71 w188 w284 w355 w612]
        tunnel: [w65 w82 w180 w294 w355 w612] -> w39
        tunnel: [dbl[][] [] w84 w181 w285 w313 w608] -> w42
        tunnel: w41 -> [_ w84 w181 w285 w345 w608]
        tunnel: w40 -> [w59 _ _ _ _ _]
        tunnel: [w64 w82 w180 w283 w337 w604] -> w37
        tunnel: w36 -> [w64 _ _ w283 w337 w604]
        tunnel: [w57 State."Preprocessing" ("Enum") State."Preprocessing" ("Enum") State."Compute AR/MA Coeffs" ("Enum") State."Get Spectrum" ("Enum") w593] -> w32
        tunnel: [_ w73 _ w277 w295 w590] -> w31
        tunnel: w30 -> [_ w72 _ w277 w295 w590]
        frame "Initialize" {
          w60 = 0.0 ("Critical Frequency [Hz]")
          w62 = waveform(dbl)[] [] ("History Data")
          w58 = dbl[] [] ("Array - Numeric")
          # "Reset all data values"
          # "Resets the graphs"
          # "Initialize the current run and indicate whether this is a simulation or not"
          n27 = local write "Damping Ratios (%)"(w58) -> ()
          n28 = To Double Precision Complex(1:w58) -> (0:w63:cdb[])
          n29 = local write "Natural Frequencies"(w58) -> ()
          n30 = local write "Frequency[Hz]"(w58) -> ()
          n31 = local write "Damping Ratio [%]"(w58) -> ()
          n32 = local write "Complex Poles"(w63) -> ()
          n33 = local write "Mean Damping [%]"(w58) -> ()
          n34 = local write "Std of Damping"(w58) -> ()
          n35 = local write "Poles"(w63) -> ()
          n36 = invoke on="Spectrogram" class="3D Surface (strict)" method="Clean Data.vi"() -> ()  [unwired: 3 in, 3 out]
          n37 = property on="Preprocessed data" class="WFChart (strict)"("History Data"=w62) -> ()  [unwired: 2 in, 2 out]
          n38 = property on="Real-time data" class="WFChart (strict)"("History Data"=w62) -> ()  [unwired: 2 in, 2 out]
          n39 = local write "Critical Frequency [Hz]"(w60) -> ()
          n40 = local write "Estimated Complex Plane"(cluster{"Array":dbl[], "Array 2":dbl[]} {"Array"=[], "Array 2"=[]} ("Cluster")) -> ()
          n41 = local write "Critical Damping [%]"(w60) -> ()
          n42 = case shown="True" w59 {
            tunnel: [State."Read Real Data" ("Enum") State."Read Simulated Data" ("Enum")] -> w57
            frame False {
              w67 = T8."Disabled and Grayed Out" ("Disabled")
              # "This is NOT a simulation"
              n43 = property on="Input Frequency (Hz)" class="DigNum (strict)"("DisabledEnum"=w67) -> ()  [unwired: 2 in, 2 out]
              n44 = property on="Input Damping Ratio (%)" class="DigNum (strict)"("DisabledEnum"=w67) -> ()  [unwired: 2 in, 2 out]
              n45 = property on="Simulation Method" class="Enum (strict)"("DisabledEnum"=w67) -> ()  [unwired: 2 in, 2 out]
              n46 = property on="Input Zeros" class="Arr (strict)"("DisabledEnum"=w67) -> ()  [unwired: 2 in, 2 out]
              n47 = property on="Input Poles" class="Arr (strict)"("DisabledEnum"=w67) -> ()  [unwired: 2 in, 2 out]
            }
            frame True {
              # "This is a simulation"
              n48 = property on="Real-time data" class="WFChart (strict)"("Visible"=TRUE) -> ()  [unwired: 2 in, 2 out]
              n49 = property on="Simulation Method" class="Enum (strict)"("DisabledEnum"=T8."Disabled" ("Disabled")) -> ()  [unwired: 2 in, 2 out]
            }
          }
          "Simulation" <- w59
        }
        frame "Read Real Data" {
          # "Reads data provided from an input containing Real Data; Puts Waveform, \nParcel length, Sampling freq, AR order and MA order into Data Cluster \n            --- Only runs if the current run is NOT a simulation ---"
          n50 = case shown="\"Read from CSV File\"" "Test Method" {
            tunnel: [w102 w115] -> w80
            tunnel: [w97 w114] -> w77
            tunnel: [w95 w113] -> w79
            tunnel: [w92 w108] -> w75
            tunnel: [_ w104] -> w73
            tunnel: w72 -> [_ w103]
            frame "Use PRL Data" {
              (unwired) T8."Disabled and Grayed Out" ("Disabled")
              # "Index is based on channel selector\nvalues"
              n51 = call <vilib>:"PRL Read Buffer .vi"("Get All Signals"=TRUE, "Get Full Buffer"=TRUE) -> ("Analog Signals"=w96:sgl[][], "Phasor Signals"=w93:csg[][], "Timestamp"=w102:timestamp[])  [unwired: 4 in, 3 out]
              n52 = Index Array "Index Array"(array=w96, index (col)=0 ("disabled index (col)")) -> (element=w95:sgl[])  [unwired: 1 in]
              n53 = Index Array "Index Array"(array=w93, index (col)=1 ("disabled index (col)")) -> (element=w92:csg[])  [unwired: 1 in]
              n54 = Index Array "Index Array"(array=w93, index (col)=0 ("disabled index (col)")) -> (element=w97:csg[])  [unwired: 1 in]
            }
            frame "Read from CSV File" {
              n55 = First Call?() -> (First Call?: T/F=w106:bool)
              n56 = case shown="True" w106 {
                tunnel: [w117 w119] -> w104
                tunnel: [w116 w118] -> w107
                tunnel: "CSV Reader Inputs" -> [w116 w118]
                tunnel: w103 -> [w117 _]
                frame False {
                }
                frame True {
                  n57 = call "CSV Reader.vi"("CSV Reader Inputs"=w118) -> ("Terminals"=w119:T14[])  [unwired: 9 in, 1 out]
                }
              }
              n58 = for {
                tunnel: w104 -> [w130] mode=indexing
                tunnel: "Terminal ID" -> [w131]
                tunnel: [w130] -> w111
                tunnel: w107 -> [w129]
                stop <- w126 stop-if-true
                n59 = Unbundle By Name(w129) -> ("OGE Type"=w125:enum16{"WAN OGE", "OGnE"})
                n60 = Unbundle By Name(w130) -> ("Terminal ID"=w132:dbl)
                n61 = Equal?(x=w132, y=w131) -> (x = y?=w128:bool)
                n62 = Equal?(x=w125, y=enum16{"WAN OGE", "OGnE"}."WAN OGE" ("OGE Type")) -> (x = y?=w127:bool)
                n63 = Or(x=w127, y=w128) -> (x .or. y?=w126:bool)
              }
              n64 = for {
                tunnel: w104 -> [w121] mode=indexing
                tunnel: "Terminal ID 2 (Phase Comparison)" -> [w122]
                tunnel: [w121] -> w109
                stop <- w120 stop-if-true
                n65 = Unbundle By Name(w121) -> ("Terminal ID"=w123:dbl)
                n66 = Equal?(x=w123, y=w122) -> (x = y?=w120:bool)
              }
              n67 = Unbundle By Name(w111) -> ("Timestamps"=w115:timestamp[], "Phasor Data"=w114:cdb[], "Analog Data"=w113:dbl[])
              n68 = Unbundle By Name(w109) -> ("Phasor Data"=w108:cdb[])
            }
          }
          n69 = case shown="\"Phase\"" "Signal Selection" {
            tunnel: [w133 w143 w145 w147 w149] -> w76
            tunnel: w77 -> [w141 _ w146 w148 w150]
            tunnel: w79 -> [_ w142 _ _ _]
            tunnel: w75 -> [w136 _ _ _ _]
            frame "Phase" {
              w137 = 0 items=["radian in, radian out", "radian in, degree out", "degree in, degree out", "degree in, radian out"] ("phase unit")
              w140 = 0 items=["radian in, radian out", "radian in, degree out", "degree in, degree out", "degree in, radian out"] ("phase unit")
              n70 = Complex To Polar(r * e^(i*theta)=w136) -> (theta=w138:dbl[])  [unwired: 1 out]
              n71 = Complex To Polar(r * e^(i*theta)=w141) -> (theta=w139:dbl[])  [unwired: 1 out]
              n72 = call <vilib>:"Unwrap Phase.vi"("phase unit"=w137, "Phase"=w138) -> ("Unwrapped Phase"=w134:dbl[])  [unwired: 8 in, 1 out]
              n73 = call <vilib>:"Unwrap Phase.vi"("phase unit"=w140, "Phase"=w139) -> ("Unwrapped Phase"=w135:dbl[])  [unwired: 8 in, 1 out]
              n74 = Subtract(x=w135, y=w134) -> (x-y=w133:dbl[])
            }
            frame "Analog" {
              n75 = To Double Precision Float(number=w142) -> (double precision float=w143:dbl[])
            }
            frame "Mag", Default {
              n76 = Complex To Polar(r * e^(i*theta)=w146) -> (r=w144:dbl[])  [unwired: 1 out]
              n77 = To Double Precision Float(number=w144) -> (double precision float=w145:dbl[])
            }
            frame "Imaginary Component" {
              n78 = Complex To Re/Im(x + iy=w148) -> (y=w147:dbl[])  [unwired: 1 out]
            }
            frame "Real Component" {
              n79 = Complex To Re/Im(x + iy=w150) -> (x=w149:dbl[])  [unwired: 1 out]
            }
          }
          n80 = local read "Sampling Frequency (Hz)"() -> (w88:dbl)
          n81 = Reciprocal(x=w88) -> (1/x=w91:dbl)
          n82 = local read "MA Order"() -> (w87:i32)
          n83 = local read "AR Order"() -> (w89:i32)
          n84 = Index Array "Index Array"(array=w80, index=0) -> (element=w85:timestamp)
          n85 = Array Size(array=w76) -> (size(s)=w81:i32)
          n86 = Bundle By Name("t0"=w85, "dt"=w91, "Y"=w76) -> (w90:waveform(dbl))  [unwired: 1 in]
          n87 = Bundle By Name(cluster=w71, "Waveform"=w90, "Parcel Length"=w81, "Sampling Frequency"=w88, "AR Order"=w89, "MA Order"=w87) -> (w82:T9)
        }
        frame "Read Simulated Data" {
          w158 = "H"
          # "Enter data into the Data cluster"
          n88 = case shown="\"Use Input Poles/Zeroes\"" "Simulation Method" {
            tunnel: [dbl[] [1.0] ("Array") w210] -> w156
            tunnel: [w204 w212] -> w155
            frame "Use Input Frequency/D.R." {
              w189 = T8."Disabled and Grayed Out" ("Disabled")
              n89 = Multiply(x=2.0 ("y"), y=3.141592653589793) -> (x*y=w206:dbl)
              n90 = Multiply(x="Input Frequency (Hz)", y=w206) -> (x*y=w202:dbl)
              n91 = Divide(x="Input Damping Ratio (%)", y=100.0) -> (x/y=w192:dbl)
              n92 = Square(x=w202) -> (x^2=w201:dbl)
              n93 = Square(x=w192) -> (x^2=w195:dbl)
              n94 = Subtract(x=1.0 ("standard deviation"), y=w195) -> (x-y=w194:dbl)
              n95 = Divide(x=w201, y=w194) -> (x/y=w193:dbl)
              n96 = Square Root(x=w193) -> (sqrt(x)=w197:dbl)
              n97 = Multiply(x=w197, y=w192) -> (x*y=w198:dbl)
              n98 = Multiply(x=w198, y=2.0) -> (x*y=w200:dbl)
              n99 = property on="Input Zeros" class="Arr (strict)"("DisabledEnum"=w189) -> ()  [unwired: 2 in, 2 out]
              n100 = Build Array(w193, w200, 1.0 ("standard deviation")) -> (w204:dbl[])
              n101 = property on="Input Poles" class="Arr (strict)"("DisabledEnum"=w189) -> ()  [unwired: 2 in, 2 out]
            }
            frame "Use Input Poles/Zeroes" {
              w214 = T8."Disabled and Grayed Out" ("Disabled")
              n102 = mathscript code="[num, den] = zpk_to_tf(zeros, poles, 1)"("zeros"="Input Zeros", "poles"="Input Poles") -> ("num"=w211:dbl[], "den"=w213:dbl[])  [unwired: 1 in, 1 out]
              n103 = property on="Input Frequency (Hz)" class="DigNum (strict)"("DisabledEnum"=w214) -> ()  [unwired: 2 in, 2 out]
              n104 = property on="Input Damping Ratio (%)" class="DigNum (strict)"("DisabledEnum"=w214) -> ()  [unwired: 2 in, 2 out]
              n105 = Reverse 1D Array(array=w213) -> (reversed array=w212:dbl[])
              n106 = Reverse 1D Array(array=w211) -> (reversed array=w210:dbl[])
            }
          }
          n107 = call <vilib>:"Gaussian White Noise.vi"("standard deviation"=10.0, "samples"="Parcel Length (Simulation)") -> ("Gaussian noise pattern"=w177:dbl[])  [unwired: 8 in, 1 out]
          n108 = Reshape Array "Reshape Array"(w177, 1 ("dimension size"), 30000 ("dimension size")) -> (w176:dbl[][])
          n109 = call-poly <vilib>:"CD Construct Transfer Function Model.vi"("Denominator"=w155, "Numerator"=w156) -> ("error out"=w159:errorcluster, "Transfer Function Model"=w161:T15)  [unwired: 8 in]
          n110 = call-poly <vilib>:"CD Set Names to Model.vi"("Model Name"=w158, "Transfer Function Model In"=w161, "error in (no error)"=w159) -> ("Model Out"=w154:T15, "error out"=w160:errorcluster)  [unwired: 11 in]
          n111 = call-poly <vilib>:"CD Draw Transfer Function Equation.vi"("Function Name (empty)"=w158, "error in (no error)"=w160, "Transfer Function Model"=w154) -> ("error out"=w157:errorcluster, "Equation"=→"Input Transfer Function":picture)  [unwired: 6 in, 1 out]
          n112 = call-poly <vilib>:"CD Linear Simulation.vi"("Delta t"=0.02, "error in (no error)"=w157, "Inputs"=w176, "Transfer Function Model"=w154) -> ("Simulation Data"=w175:T18)  [unwired: 5 in, 2 out]
          n113 = Unbundle By Name(w175) -> ("Outputs Data"=w172:dbl[][][])
          n114 = call-poly <vilib>:"CD Damping Ratio and Natural Frequency.vi"("Transfer Function Model"=w154) -> ("Poles"=→"Poles":cdb[], "Natural Frequencies"=→"Natural Frequencies":dbl[], "Damping Ratios"=w166:dbl[])  [unwired: 7 in, 1 out]
          n115 = To Double Precision Float(number=100 ("length")) -> (double precision float=w163:dbl)
          n116 = Multiply(x=w163, y=w166) -> (x*y=→"Damping Ratios (%)":dbl[])
          n117 = Get Date/Time In Seconds() -> (seconds since 1Jan1904=w179:timestamp)
          n118 = Index Array "Index Array"(array=w172, index (dim 0)=0 ("index"), index (dim 2)=0 ("length")) -> (element=w170:dbl[])  [unwired: 1 in]
          n119 = Reciprocal(x="Sampling Frequency (Hz)") -> (1/x=w184:dbl)
          n120 = Bundle By Name("t0"=w179, "dt"=w184, "Y"=w170) -> (w185:waveform(dbl))  [unwired: 1 in]
          n121 = Bundle By Name(cluster=w188, "Waveform"=w185, "Parcel Length"="Parcel Length (Simulation)", "Sampling Frequency"="Sampling Frequency (Hz)", "AR Order"="AR Order", "MA Order"="MA Order") -> (w180:T9)
        }
        frame "Preprocessing" {
          # "New Waveform and Frequency"
          # "Detrend the transfer function, pass it through a LPF, then rescale it (downsample)"
          n122 = Unbundle By Name(w284) -> ("Waveform"=w286:waveform(dbl), "Sampling Frequency"=w288:dbl, "Parcel Length"=→"Parcel Length (SDK or Simulation)":i32)
          n123 = call-poly <vilib>:"WA Detrend.vi"("threshold frequency"="Detrend Cut-off Frequency (Hz)", "signal"=w286) -> ("detrended signal"=w290:waveform(dbl))  [unwired: 7 in, 2 out]
          n124 = call-poly "SI Lowpass Filter.vi"("cutoff frequency"="LPF Cut-off Frequency [Hz]", "order"="Low-Pass Filter Order", "stimulus signal in"=w290) -> ("stimulus signal out"=w289:waveform(dbl))  [unwired: 6 in, 2 out]
          n125 = To Long Integer(number="Downsampling Ratio") -> (32bit integer=w280:i32)
          n126 = call "Downsample.vi"("Divide by"=w280, "Waveform in"=w289) -> ("Waveform out"=w282:waveform(dbl))  [unwired: 9 in]
          "Preprocessed data" <- w282
          n127 = Divide(x=w288, y="Downsampling Ratio") -> (x/y=w287:dbl)
          n128 = Bundle By Name(cluster=w284, "Waveform"=w282, "Sampling Frequency"=w287) -> (w294:T9)
        }
        frame "Compute AR/MA Coeffs" {
          w353 = T20 5 items=["Zero-Order-Hold", "Tustin (Bilinear)", "Prewarp", "Forward", "Backward", "Z-Transform"] ("Method")
          w356 = u16 0 items=["Yule-Walker", "High order AR", "Polynomial"] ("method")
          # "maybe add tsa modal parametric modeling??"
          # "Convert back into s-domain"
          # "Eliminates the poles that have negative/0 complex component,\nand eliminates duplicate frequencies/damping ratios and those \noutside of the bounds (as per the lower/upper values)"
          n129 = control-ref of="Estimated Complex Plane"() -> (w347:refnum<vi>)
          n130 = Unbundle By Name(w355) -> ("Waveform"=w354:waveform(dbl), "AR Order"=w352:i32, "MA Order"=w316:i32, "Sampling Frequency"=w314:dbl)
          n131 = property class="XYGraph (strict)"(reference=w347, "BG Color"=u32 16448250 ("Color Box")) -> ()  [unwired: 1 in, 2 out]
          n132 = Bundle("AR Order"=w352, "MA Order"=w316) -> (w351:cluster{"AR Order":i32, "MA Order ":i32})  [unwired: 1 in]
          n133 = Reciprocal(x=w314) -> (1/x=w315:dbl)
          n134 = call-poly <vilib>:"TSA ARMA Modeling.vi"("ARMA order"=w351, "method"=w356, "Xt"=w354) -> ("error out"=w297:errorcluster, "MA coefficients"=w303:dbl[], "AR coefficients"=w306:dbl[])  [unwired: 5 in, 1 out]
          n135 = Reverse 1D Array(array=w306) -> (reversed array=w331:dbl[])
          n136 = Reverse 1D Array(array=w303) -> (reversed array=w332:dbl[])
          n137 = call-poly <vilib>:"CD Construct Transfer Function Model.vi"("Sampling Time (s)"=w315, "error in (no error)"=w297, "Denominator"=w331, "Numerator"=w332) -> ("error out"=w299:errorcluster, "Transfer Function Model"=w302:T15)  [unwired: 6 in]
          n138 = call-poly <vilib>:"CD Draw Transfer Function Equation.vi"("Function Name (empty)"="   B(z) / A", "error in (no error)"=w299, "Transfer Function Model"=w302) -> ("error out"=w298:errorcluster, "Equation"=→"ARMA Transfer Function":picture)  [unwired: 6 in, 1 out]
          n139 = call-poly <vilib>:"CD Convert Discrete to Continuous.vi"("error in (no error)"=w298, "Method"=w353, "Discrete Transfer Function Model"=w302) -> ("error out"=w326:errorcluster, "Continuous Transfer Function Model"=w320:T15)  [unwired: 7 in]
          n140 = call-poly <vilib>:"CD Convert to State-Space Model.vi"("error in (no error)"=w326, "Realization Type"=enum16{"minimum", "full"}."full", "Transfer Function Model"=w320) -> ("error out"=w319:errorcluster, "State-Space Model"=w324:T21)  [unwired: 7 in]
          n141 = call-poly <vilib>:"CD Damping Ratio and Natural Frequency.vi"("error in (no error)"=w319, "Frequency Unit"=enum16{"Hz", "rad/s"}."Hz", "State-Space Model"=w324) -> ("Poles"=w333:cdb[], "Natural Frequencies"=w327:dbl[], "Damping Ratios"=w341:dbl[])  [unwired: 5 in, 1 out]
          n142 = To Double Precision Float(number=100 ("Numeric")) -> (double precision float=w318:dbl)
          n143 = Multiply(x=w318, y=w341) -> (x*y=w339:dbl[])
          n144 = mathscript code="[damp,ind]=sort(damp);\nfreq=freq(ind);\npoles=poles(ind);\n\nind=find(freq>LowF & freq<UpF & damp>LowD & damp<UpD &  imag(poles)>=0)\ndamp=damp(ind)\nfreq=freq(ind);\npoles=poles(ind);"("damp"=w339, "freq"=w327, "poles"=w333, "LowF"="Lower Frequency [Hz]", "UpF"="Upper Frequency [Hz]", "LowD"="Lower Damping [%]", "UpD"="Upper Damping [%]") -> ("poles"=w323:cdb[], "freq"=w305:dbl[], "damp"=w304:dbl[])  [unwired: 1 in, 1 out]
          "Complex Poles" <- w323
          "Frequency[Hz]" <- w305
          "Damping Ratio [%]" <- w304
          n145 = Build Array (concatenate) "Build Array"(w304, w345) -> (w313:dbl[][])
          n146 = local read "Length of Spectra [s]"() -> (w340:dbl)
          n147 = Complex To Re/Im(x + iy=w323) -> (x=w350:dbl[], y=w349:dbl[])
          n148 = Bundle(w350, w349) -> (→"Estimated Complex Plane":cluster{dbl[], dbl[]})  [unwired: 1 in]
          n149 = Array Subset "Array Subset"(array=w313, index (row)=0 ("index"), length (row)=w340, index (col)=0 ("index"), length (col)="Number of critical modes") -> (w312:dbl[][])
          n150 = Transpose 2D Array(2D array=w312) -> (transposed array=→"Damping ratio evolution":dbl[][])
          n151 = for {
            N: "Number of critical modes" -> [_]
            tunnel: w313 -> [w372]
            tunnel: [w370] -> w338 mode=indexing
            tunnel: [w369] -> w311 mode=indexing
            i -> [w368]
            # "Take Std. Deviation and Mean\nof Damping Ratios"
            n152 = Index Array "Index Array"(array=w372, index (col)=w368) -> (element=w371:dbl[])  [unwired: 1 in]
            n153 = call <vilib>:"Std Deviation and Variance.vi"("X"=w371, "Weighting (Sample)"=enum16{"Sample", "Population"}."Sample") -> ("mean"=w370:dbl, "standard deviation"=w369:dbl)  [unwired: 1 out]
          }
          "Std of Damping" <- w311
          "Mean Damping [%]" <- w338
          n154 = call "smiley.vi"("std threshold"="Std Threshold", "damp"=w311) -> ("Array"=w336:picture[])  [unwired: 9 in]
          n155 = Index Array(array=w305, index=0) -> (element=→"Critical Frequency [Hz]":dbl)
          n156 = for {
            tunnel: w336 -> [w357] mode=indexing
            i -> [w358]
            n157 = case shown="0, Default" w358 {
              tunnel: w357 -> [w359 w360 w361 w362 w363 w364 w365 w366 w367]
              frame 0, Default {
                "Picture 1" <- w359
              }
              frame 1 {
                "Picture 2" <- w360
              }
              frame 2 {
                "Picture 3" <- w361
              }
              frame 3 {
                "Picture 4" <- w362
              }
              frame 4 {
                "Picture 5" <- w363
              }
              frame 5 {
                "Picture 6" <- w364
              }
              frame 6 {
                "Picture 7" <- w365
              }
              frame 7 {
                "Picture 8" <- w366
              }
              frame 8 {
                "Picture 9" <- w367
              }
            }
          }
          n158 = Index Array(array=w304, index=0 ("length")) -> (element=→"Critical Damping [%]":dbl)
        }
        frame "Get Spectrum" {
          w614 = u16 0 items=["Yule-Walker", "High order AR", "Polynomial"] ("method")
          # "Continue to read the data"
          n159 = local read "Refresh Rate [s]"() -> (w599:i32)
          n160 = Unbundle By Name(w612) -> ("Waveform"=w624:waveform(dbl), "AR Order"=w627:i32, "MA Order"=w626:i32)
          n161 = Bundle("AR Order"=w627, "MA Order"=w626) -> (w625:cluster{"AR Order":i32, "MA Order ":i32})  [unwired: 1 in]
          n162 = call-poly <vilib>:"TSA ARMA Spectrum.vi"("dB on? (T)"="dB Scale", "ARMA order"=w625, "method"=w614, "Xt"=w624) -> ("PSD"=w613:cluster{"f0":dbl, "df":dbl, "S(f)":dbl[]})  [unwired: 5 in, 2 out]
          "Spectrum" <- w613
          n163 = To Double Precision Float(number=w599) -> (double precision float=w600:dbl)
          n164 = Unbundle By Name(w613) -> ("f0"=w622:dbl, "df"=w621:dbl, "S(f)"=w618:dbl[])
          n165 = Quotient & Remainder(x="Length of Spectra [s]", y=w600) -> (floor(x/y)=w602:dbl)  [unwired: 1 out]
          n166 = Increment(x=w602) -> (x+1=w601:dbl)
          n167 = for {
            tunnel: w618 -> [_] mode=indexing
            tunnel: w622 -> [w631]
            tunnel: w621 -> [w633]
            tunnel: [w630] -> w610 mode=indexing
            i -> [w634]
            n168 = Decrement(x=w634) -> (x-1=w628:i32)
            n169 = To Double Precision Float(number=w628) -> (double precision float=w629:dbl)
            n170 = Multiply(x=w633, y=w629) -> (x*y=w632:dbl)
            n171 = Add(x=w631, y=w632) -> (x+y=w630:dbl)
          }
          n172 = feedback #1(dbl[] [] ("XX")) -> (w620:dbl[])
          n173 = feedback #2(0.0 ("i")) -> (w623:dbl)
          n174 = feedback #3(0.0 ("TDold")) -> (w606:dbl)
          n175 = feedback #4(dbl[][] [] ("Array")) -> (w616:dbl[][])
          n176 = mathscript code="if (TDold ~=TimeDiff)\ni=0\nend\nif i>Limit\nXX=XX(i-Limit+1:i);\ni=Limit;\nend\nif i==Limit\nArray=Array(2:i,:);\nArray(i,:)=Data(:);\nelse\ni=i+1\nArray(i,:)=Data(:);\nXX(i)=0;\n\nif i==1\nXX(1)=0;\nelse\nXX(1:i-1)=XX(1:i-1)-TimeDiff\nXX(i)=0\nend\nend\n\nTDold=TimeDiff;"("Data"=w618, "Array"=w616, "i"=w623, "Limit"=w601, "XX"=w620, "TimeDiff"=w599, "TDold"=w606) -> ("Array"=w609:dbl[][], "i"=w597:dbl, "XX"=w607:dbl[], "TDold"=w594:i32)  [unwired: 1 in, 1 out]
          n177 = feedback-in #1(w607) -> ()
          n178 = feedback-in #2(w597) -> ()
          n179 = To Double Precision Float(number=w594) -> (double precision float=w595:dbl)
          n180 = feedback-in #3(w595) -> ()
          n181 = feedback-in #4(w609) -> ()
          n182 = call-poly <vilib>:"Plot Helper.vi"("z matrix"=w609, "y vector"=w610, "x vector"=w607) -> ("3D Plot lvclass Array out"=→"Spectrogram":refnum<class "3D Plot Datatype.lvclass">[])  [unwired: 3 in, 5 out]
          n183 = local read "Simulation"() -> (w611:bool)
          n184 = Select(t=State."Read Simulated Data" ("Enum"), s=w611, f=State."Read Real Data" ("Enum")) -> (s? t:f=w593:T10)
        }
      }
      n185 = local read "Refresh Rate [s]"() -> (w45:i32)
      n186 = Multiply(x=w45, y=1000) -> (x*y=w34:i32)
      n187 = To Double Precision Float(number=w34) -> (double precision float=w35:dbl)
      n188 = Divide(x=w35, y=4.0) -> (x/y=w46:dbl)
      n189 = To Quad Integer(1:w46) -> (0:w43:i64)
      n190 = Not Equal?(x=w43, y=w50) -> (x != y?=w49:bool)
      n191 = Or(x=w49, y="stop") -> (x .or. y?=w51:bool)
      n192 = Unbundle By Name(w37) -> ("Waveform"=→"Real-time data":waveform(dbl))
      n193 = node-c288() -> ()  [unwired: 1 in, 1 out]
    }
    n194 = node-c288(w18) -> ()  [unwired: 1 out]
  }
